vi "Configure.vi"(8 "error in":errorcluster, 10 "name":string, 11 "CRDS in":refnum<class "CRDS.lvclass">) -> (0 "error out":errorcluster, 3 "CRDS out":refnum<class "CRDS.lvclass">)   [LabVIEW 2014, in "CRDS Lib.lvlib" / "CRDS.lvclass"]
doc: "Configure the instrument class. If there is no config file specified, an error"
uses:
  CRDS.lvclass
  Data/Main/CRDS Data.lvclass
  General/Math/Fit Exponential Class/Children/LRS/LRS.lvclass
  General/Math/Fit Exponential Class/Fit Exponential.lvclass/Fit Exponential.ctl
  Instrument/Instrument.lvclass/Instrument.ctl
  Session APIs/File Access/Config Data/Config Data.lvclass/Config Data.ctl
  Data/Cell/CRDS Cell Data.lvclass
  Data/Data.lvclass/Data.ctl
  Data/Cell/CRDS Cell Data.lvclass/CRDS Cell Data.ctl
  Cell/CRDS Cell.lvclass/CRDS Cell.ctl
  Data/Write Data ID.vi
  Data/Cell/Write Ncell.vi
  Data/Cell/Write Write RD_.vi
  Cell/Write ExpFit.vi
  Cell/Write Data.vi
  General/Math/Fit Exponential Class/Write Get A_B.vi
  Instrument/Read Cfg Session.vi
  Session APIs/File Access/Config Data/Accessors/Read Ref.vi
  Instrument/Write Data OK_.vi
  Instrument/Write Data.vi
  Read Cells.vi
  <vilib>/Utility/config.llb/Read Key (I32).vi
  <vilib>/Utility/config.llb/Read Key (Boolean).vi
  Session APIs/File Access/Config Data/Read Array/Read DBL Array.vi
  Session APIs/File Access/Config Data/Read Array/Read String Array.vi
  Cell/Write lambda.vi
  Cell/Write optTimeConst.vi
  Data/Main/Write CellData.vi
  Write Cells.vi
  Instrument/Instrument.lvclass
  Cell/CRDS Cell.lvclass
  Session APIs/File Access/Config Data/Config Data.lvclass
  <vilib>/Utility/config.llb/NI_LVConfig.lvlib
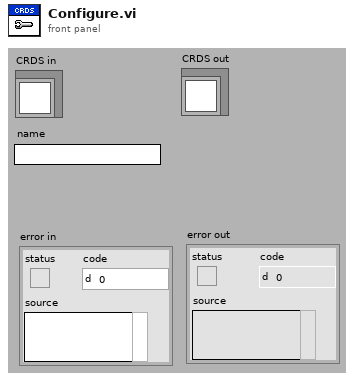
[diagram p1: front panel]
types:
  T1 = typedef "Config Data.lvclass/Config Session.ctl" = refnum<data-value>
  T2 = typedef "NI_LVConfig.lvlib/Config Data RefNum.ctl" = refnum<k1>
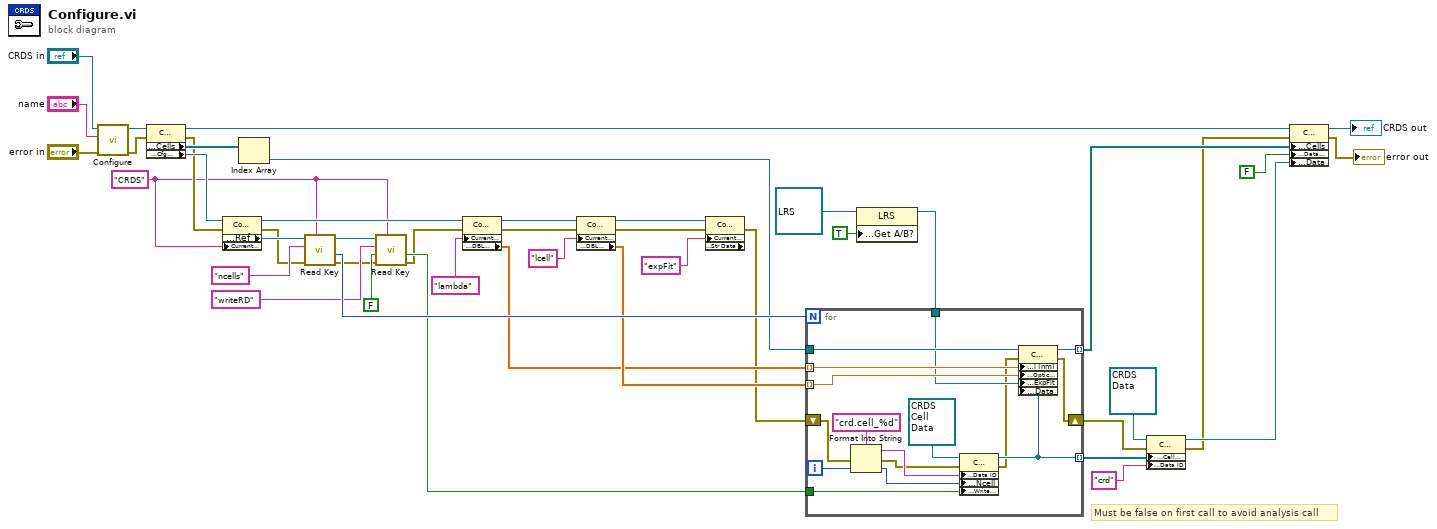
[diagram p0: block diagram]
diagram:
  w4 = "CRDS" ("section")
  # "Must be false on first call to avoid analysis call"
  n1 = call-parent "Configure.vi"("error in"="error in", "name"="name", "Instrument in"="CRDS in") -> ("error out"=w12:errorcluster, "Instrument out"=w42:refnum<class "CRDS.lvclass">)  [unwired: 7 in]
  n2 = property class="CRDS"(reference=w42, error in=w12) -> (reference out=w28:refnum<class "CRDS.lvclass">, error out=w9:errorcluster, "Data Access:Cells"=w10:refnum<class "CRDS Cell.lvclass">[], "Accessors:Cfg Session"=w11:T1)
  n3 = property class="Config Data"(reference=w11, error in=w9, "Current Section"=w4) -> (reference out=w40:T1, error out=w5:errorcluster, "Accessors:Ref"=w6:T2)
  n4 = Index Array(array=w10) -> (element=w32:refnum<class "CRDS Cell.lvclass">)  [unwired: 1 in]
  n5 = call-poly <vilib>:"Read Key.vi"("section"=w4, "error in (no error)"=w5, "key"="ncells", "refnum"=w6) -> ("error out"=w7:errorcluster, "value"=w33:i32, "refnum out"=w8:T2)  [unwired: 4 in, 1 out]
  n6 = call-poly <vilib>:"Read Key.vi"("section"=w4, "error in (no error)"=w7, "default value"=FALSE, "key"="writeRD", "refnum"=w8) -> ("error out"=w3:errorcluster, "value"=w16:bool)  [unwired: 3 in, 2 out]
  n7 = property class="Config Data"(reference=w40, error in=w3, "Current Key"="lambda") -> (reference out=w38:T1, error out=w37:errorcluster, "Read Array Data:DBL Data"=w30:dbl[])
  n8 = property class="Config Data"(reference=w38, error in=w37, "Current Key"="lcell") -> (reference out=w36:T1, error out=w35:errorcluster, "Read Array Data:DBL Data"=w31:dbl[])
  n9 = property class="Config Data" props=["Current Key", "Read Array Data:Str Data"](reference=w36, error in=w35, "Current Key"="expFit") -> (error out=w20:errorcluster)  [unwired: 2 out]
  n10 = property class="LRS"(reference=refnum<class "LRS.lvclass"> refnum ("Exponential Fit Lib:LRS"), "Accessors:Get A/B?"=TRUE ("Get A/B?")) -> (reference out=w13:refnum<class "LRS.lvclass">)  [unwired: 1 in, 1 out]
  n11 = for {
    N: w33 -> [_]
    tunnel: w32 -> [w60]
    tunnel: w31 -> [w59] mode=indexing
    tunnel: w30 -> [w58] mode=indexing
    tunnel: [w56] -> w27 mode=indexing
    tunnel: [w51] -> w22 mode=indexing
    tunnel: w13 -> [w55]
    tunnel: w16 -> [w49]
    shift-right: [w57] -> w2
    shift-left: w20 -> [w48]
    i -> [w50]
    n12 = Format Into String(format string="crd.cell_%d", error in=w48, w50) -> (resulting string=w52:string, error out=w47:errorcluster)  [unwired: 1 in]
    n13 = property class="CRDS Cell"(reference=refnum<class "CRDS Cell Data.lvclass"> refnum ("CRDS Cell"), error in=w47, "Accessors:Data ID"=w52, "Data Access:Ncell"=w50, "Data Access:Write RD_"=w49) -> (reference out=w51:refnum<class "CRDS Cell Data.lvclass">, error out=w46:errorcluster)
    n14 = property class="CRDS Cell"(reference=w60, error in=w46, "Data Access:l (nm)"=w58, "Data Access:Optical Time Constant"=w59, "Data Access:ExpFit"=w55, "Data Access:Data"=w51) -> (reference out=w56:refnum<class "CRDS Cell.lvclass">, error out=w57:errorcluster)
  }
  n15 = property class="CRDS"(reference=refnum<class "CRDS Data.lvclass"> refnum ("CRDS"), error in=w2, "Accessors:Cell Data"=w22, "Accessors:Data ID"="crd" ("Data ID")) -> (reference out=w21:refnum<class "CRDS Data.lvclass">, error out=w1:errorcluster)
  n16 = property class="CRDS"(reference=w28, error in=w1, "Data Access:Cells"=w27, "Accessors:Data OK_"=FALSE ("Data Ready?"), "Accessors:Data"=w21) -> (reference out=→"CRDS out":refnum<class "CRDS.lvclass">, error out=→"error out":errorcluster)
